vi "testpath5.vi"() -> (4 "Trajectory":T1[](array[typedef])=[{"t"=0.0, "velocity"=0.0, "acceleration"=1.0, "pose"={"Translation2d"={"x"=3.0, "y"=3.0}, "Rotation2d"={"Theta"=0.0}}, "curvature"=0.0}, {"t"=0.48107866498249907, "velocity"=0.48107866498249907, "acceleration"=1.0, "pose"={"Translation2d"={"x"=3.1157180698455615, "y"=3.0002504867135467}, "Rotation2d"={"Theta"=0.006427363502563971}}, "curvature"=0.1089996880264415}, {"t"=0.678323361711993, "velocity"=0.678323361711993, "acceleration"=1.0, "pose"={"Translation2d"={"x"=3.230048850761391, "y"=3.001918683513517}, "Rotation2d"={"Theta"=0.024668187651407807}}, "curvature"=0.20964722526020957}, {"t"=0.8269742084287445, "velocity"=0.8269742084287445, "acceleration"=1.0, "pose"={"Translation2d"={"x"=3.3418489753345284, "y"=3.006195017751254}, "Rotation2d"={"Theta"=0.05364254472795485}}, "curvature"=0.3088358096240247}, {"t"=0.9493182706582894, "velocity"=0.9493182706582894, "acceleration"=0.9999999999999989, "pose"={"Translation2d"={"x"=3.4502251031388798, "y"=3.0140362049070544}, "Rotation2d"={"Theta"=0.09263700599383605}}, "curvature"=0.4097816878257488}, {"t"=1.0541332693458725, "velocity"=1.0541332693458723, "acceleration"=1.0, "pose"={"Translation2d"={"x"=3.554516244600639, "y"=3.02618090481411}, "Rotation2d"={"Theta"=0.14101399179369137}}, "curvature"=0.512308874505636}, {"t"=1.1461185111358019, "velocity"=1.1461185111358017, "acceleration"=0.9999999999999989, "pose"={"Translation2d"={"x"=3.654276084863717, "y"=3.0431653778824543}, "Rotation2d"={"Theta"=0.19795363197982824}}, "curvature"=0.6126189634299863}, {"t"=1.2282728023077116, "velocity"=1.2282728023077114, "acceleration"=1.0, "pose"={"Translation2d"={"x"=3.7492553076551633, "y"=3.0653391413229074}, "Rotation2d"={"Theta"=0.2622253015840179}}, "curvature"=0.7032278829567145}, {"t"=1.3027431134377192, "velocity"=1.302743113437719, "acceleration"=1.0, "pose"={"Translation2d"={"x"=3.8393839191505923, "y"=3.092880625371018}, "Rotation2d"={"Theta"=0.33202347001519067}}, "curvature"=0.7738213581754176}, {"t"=1.3711828600338833, "velocity"=1.3711828600338831, "acceleration"=1.0, "pose"={"Translation2d"={"x"=3.9247535718396085, "y"=3.125812829511009}, "Rotation2d"={"Theta"=0.40492626492857636}}, "curvature"=0.8135150769014742}, {"t"=1.4349150919425286, "velocity"=1.4349150919425284, "acceleration"=1.0, "pose"={"Translation2d"={"x"=4.00559988839123, "y"=3.1640189786997217}, "Rotation2d"={"Theta"=0.4780242378088871}}, "curvature"=0.814144470711001}, {"t"=1.4950089576936443, "velocity"=1.495008957693644, "acceleration"=1.0000000000000024, "pose"={"Translation2d"={"x"=4.082284785519317, "y"=3.2072581795905597}, "Rotation2d"={"Theta"=0.5482106201854816}}, "curvature"=0.7731590788080065}, {"t"=1.5523180030026276, "velocity"=1.5523180030026276, "acceleration"=1.0, "pose"={"Translation2d"={"x"=4.1552787978479895, "y"=3.2551810767574345}, "Rotation2d"={"Theta"=0.6125488582787016}}, "curvature"=0.6945009614427361}, {"t"=1.6075049826736048, "velocity"=1.6075049826736048, "acceleration"=1.0, "pose"={"Translation2d"={"x"=4.225143401777062, "y"=3.307345508918708}, "Rotation2d"={"Theta"=0.6685937757440954}}, "curvature"=0.5870109054408447}, {"t"=1.661065404441924, "velocity"=1.661065404441924, "acceleration"=1.0, "pose"={"Translation2d"={"x"=4.29251333934746, "y"=3.363232165161137}, "Rotation2d"={"Theta"=0.714573100801571}}, "curvature"=0.46146389986649705}, {"t"=1.7133542364605543, "velocity"=1.7133542364605543, "acceleration"=1.0, "pose"={"Translation2d"={"x"=4.358078942106649, "y"=3.42226024116382}, "Rotation2d"={"Theta"=0.749411478919885}}, "curvature"=0.327879436774629}, {"t"=1.7646155759291982, "velocity"=1.7646155759291982, "acceleration"=-0.14069618652681756, "pose"={"Translation2d"={"x"=4.4225684549740585, "y"=3.4838030954221377}, "Rotation2d"={"Theta"=0.7726438166367136}}, "curvature"=0.19408566308886896}, {"t"=1.8158372909656526, "velocity"=1.7574088759562057, "acceleration"=-0.9999999999999976, "pose"={"Translation2d"={"x"=4.486730360106509, "y"=3.5472039054716995}, "Rotation2d"={"Theta"=0.7842865152488298}}, "curvature"=0.06554757707262261}, {"t"=1.8686030696202458, "velocity"=1.7046430973016127, "acceleration"=-0.9999999999999976, "pose"={"Translation2d"={"x"=4.551315700763633, "y"=3.611791324112289}, "Rotation2d"={"Theta"=0.7847207021181927}}, "curvature"=-0.05405445397664435}, {"t"=1.923774092685811, "velocity"=1.6494720742360478, "acceleration"=-1.0000000000000024, "pose"={"Translation2d"={"x"=4.617060405173301, "y"=3.6768951356318045}, "Rotation2d"={"Theta"=0.7746140906850375}}, "curvature"=-0.1620376344972609}, {"t"=1.9816328285536053, "velocity"=1.5916133383682531, "acceleration"=-0.9999999999999977, "pose"={"Translation2d"={"x"=4.684667610397049, "y"=3.741861912030208}, "Rotation2d"={"Theta"=0.7548841593229793}}, "curvature"=-0.2560779973743184}, {"t"=2.042535183657832, "velocity"=1.5307109832640264, "acceleration"=-1.0, "pose"={"Translation2d"={"x"=4.754789986195503, "y"=3.8060706692434647}, "Rotation2d"={"Theta"=0.7266900570486102}}, "curvature"=-0.3338915791528804}, {"t"=2.10694244004743, "velocity"=1.4663037268744283, "acceleration"=-1.0, "pose"={"Translation2d"={"x"=4.828012058893801, "y"=3.8689485233674916}, "Rotation2d"={"Theta"=0.6914332386010009}}, "curvature"=-0.39327428373518936}, {"t"=2.175457895843941, "velocity"=1.3977882710779173, "acceleration"=-1.000000000000001, "pose"={"Translation2d"={"x"=4.904832535247019, "y"=3.9299863468820986}, "Rotation2d"={"Theta"=0.6507460397676211}}, "curvature"=-0.4324325103085314}, {"t"=2.2488723273208384, "velocity"=1.3243738396010196, "acceleration"=-1.0, "pose"={"Translation2d"={"x"=4.9856466263055985, "y"=3.9887544248749345}, "Rotation2d"={"Theta"=0.606453056453139}}, "curvature"=-0.450438283054238}, {"t"=2.328227549017911, "velocity"=1.245018617903947, "acceleration"=-1.0, "pose"={"Translation2d"={"x"=5.070728371280769, "y"=4.044918111265431}, "Rotation2d"={"Theta"=0.5605017213985956}}, "curvature"=-0.447580511370689}, {"t"=2.414918055086827, "velocity"=1.158328111835031, "acceleration"=-1.0, "pose"={"Translation2d"={"x"=5.160212961409972, "y"=4.098253485028746}, "Rotation2d"={"Theta"=0.514872814070948}}, "curvature"=-0.4254088459788693}, {"t"=2.5108748508259513, "velocity"=1.062371316095907, "acceleration"=-0.9999999999999984, "pose"={"Translation2d"={"x"=5.254079063822289, "y"=4.148663006419709}, "Rotation2d"={"Theta"=0.4714931999649217}}, "curvature"=-0.38639049588199975}, {"t"=2.61893753775615, "velocity"=0.9543086291657085, "acceleration"=-1.0, "pose"={"Translation2d"={"x"=5.352131145403863, "y"=4.196191173196768}, "Rotation2d"={"Theta"=0.4321767854993178}}, "curvature"=-0.33325947480572066}, {"t"=2.743710613045412, "velocity"=0.8295355538764468, "acceleration"=-1.0000000000000004, "pose"={"Translation2d"={"x"=5.453981796663327, "y"=4.241040176845926}, "Rotation2d"={"Theta"=0.3986147043565599}}, "curvature"=-0.2682313688562159}, {"t"=2.893946469408784, "velocity"=0.6792996975130746, "acceleration"=-1.0000000000000002, "pose"={"Translation2d"={"x"=5.5590340555972295, "y"=4.283585558804693}, "Rotation2d"={"Theta"=0.3724265151781381}}, "curvature"=-0.1922294145483505}, {"t"=3.09198653643674, "velocity"=0.4812596304851187, "acceleration"=-0.9999999999999999, "pose"={"Translation2d"={"x"=5.666463731555449, "y"=4.324391866686028}, "Rotation2d"={"Theta"=0.35527729936540964}}, "curvature"=-0.10414472092652606}, {"t"=3.5732461669218587, "velocity"=0.0, "acceleration"=-0.9999999999999999, "pose"={"Translation2d"={"x"=5.775201729106637, "y"=4.364228310502283}, "Rotation2d"={"Theta"=0.3490658503988617}}, "curvature"=-4.0144373191817764e-15}], 6 "Reverse Path?":bool)   [LabVIEW 2019]
uses:
  AutonBuilder/Typedef/Data Point.ctl
  <vilib>/Rock Robotics/WPI/ThirdParty/WPILib Extensions/Trajectory/Typedef/Trajectory State.ctl
  <vilib>/Rock Robotics/WPI/ThirdParty/WPILib Extensions/Geometry/Typedef/Pose2d.ctl
  <vilib>/Rock Robotics/WPI/ThirdParty/WPILib Extensions/Geometry/Typedef/Translation2d.ctl
  <vilib>/Rock Robotics/WPI/ThirdParty/WPILib Extensions/Geometry/Typedef/Rotation2d.ctl
panel:
  out "Total Time (s)":dbl=3.5732461669218587
  out "Graph":cluster{dbl[], dbl[]}[](graph)=[{[2.8, 3.5, 3.5, 2.8, 2.8], [3.3, 3.3, 2.7, 2.7, 3.3]}, {[3.0, 5.775201729106628], [3.0, 4.364228310502283]}, {[3.0, 3.1157180698455615, 3.230048850761391, 3.3418489753345284, 3.4502251031388798, 3.554516244600639, 3.654276084863717, 3.7492553076551633, 3.8393839191505923, 3.9247535718396085, 4.00559988839123, 4.082284785519317, 4.1552787978479895, 4.225143401777062, 4.29251333934746, 4.358078942106649, 4.4225684549740585, 4.486730360106509, 4.551315700763633, 4.617060405173301, 4.684667610397049, 4.754789986195503, 4.828012058893801, 4.904832535247019, 4.9856466263055985, 5.070728371280769, 5.160212961409972, 5.254079063822289, 5.352131145403863, 5.453981796663327, 5.5590340555972295, 5.666463731555449, 5.775201729106637], [3.0, 3.0002504867135467, 3.001918683513517, 3.006195017751254, 3.0140362049070544, 3.02618090481411, 3.0431653778824543, 3.0653391413229074, 3.092880625371018, 3.125812829511009, 3.1640189786997217, 3.2072581795905597, 3.2551810767574345, 3.307345508918708, 3.363232165161137, 3.42226024116382, 3.4838030954221377, 3.5472039054716995, 3.611791324112289, 3.6768951356318045, 3.741861912030208, 3.8060706692434647, 3.8689485233674916, 3.9299863468820986, 3.9887544248749345, 4.044918111265431, 4.098253485028746, 4.148663006419709, 4.196191173196768, 4.241040176845926, 4.283585558804693, 4.324391866686028, 4.364228310502283]}, {[3.210100833045593, 3.1163674570857056, 3.2344256753709537, 3.35331553525211, 3.4718739962834073, 3.589216747032843, 3.7046276288946096, 3.8174590354897315, 3.9270558444895305, 4.032726350135738, 4.133780565975029, 4.229632160917573, 4.319925140468959, 4.404627655819516, 4.484052485239973, 4.558804117879396, 4.629684205195804, 4.697592968594799, 4.763451147629453, 4.828150889883975, 4.8925334632275135, 4.957387175141679, 5.023457384520475, 5.0914596639663925, 5.162086733508193, 5.236000987473815, 5.3138085081716895, 5.3960169412912, 5.482985919587022, 5.574881783592683, 5.671646985644121, 5.772990350008362, 5.878400124838382], [2.7858560298454615, 2.700251189554016, 2.7019506128687616, 2.7064142345051354, 2.7148183487794215, 2.7281945374565533, 2.7474210254195457, 2.7731949106602634, 2.805977098889792, 2.8459166359909562, 2.8927816031517377, 2.9459370151908018, 3.004399135897375, 3.066959563924363, 3.13233661390307, 3.1993041831366846, 3.266770687680612, 3.3338099966047543, 3.3996627023210784, 3.4637266406223106, 3.5255478181133677, 3.584814304292968, 3.641349919042501, 3.695102727134015, 3.7461253075572944, 3.7945484598763177, 3.8405551962975846, 3.8843646164518164, 3.926233717153275, 3.966480177646331, 4.005523824676723, 4.043942085867808, 4.082536828347791]}, {[2.789899166954407, 3.1150686826054175, 3.2256720261518286, 3.330382415416947, 3.428576209994352, 3.5198157421684346, 3.603924540832824, 3.681051579820595, 3.751711993811654, 3.8167807935434785, 3.877419210807431, 3.934937410121061, 3.9906324552270203, 4.045659147734609, 4.100974193454947, 4.157353766333901, 4.215452704752313, 4.275867751618218, 4.339180253897812, 4.405969920462626, 4.476801757566584, 4.552192797249327, 4.632566733267128, 4.7182054065276455, 4.809206519103004, 4.905455755087722, 5.006617414648254, 5.112141186353377, 5.221276371220704, 5.333081809733971, 5.446421125550338, 5.559937113102537, 5.672003333374892], [3.2141439701545385, 3.300249783873077, 3.301886754158273, 3.305975800997373, 3.3132540610346872, 3.3241672721716666, 3.338909730345363, 3.3574833719855515, 3.3797841518522445, 3.405709023031062, 3.4352563542477057, 3.4685793439903176, 3.505963017617494, 3.5477314539130527, 3.5941277164192043, 3.6452162991909556, 3.7008355031636633, 3.7605978143386447, 3.8239199459035, 3.8900636306412983, 3.958176005947048, 4.027327034193961, 4.0965471276924825, 4.1648699666301825, 4.2313835421925745, 4.295287762654543, 4.355951773759907, 4.412961396387602, 4.46614862924026, 4.515600176045521, 4.561647292932663, 4.604841647504248, 4.645919792656775]}]
  in  "Data Points":T5[](array[typedef])=[{"X"=3.0, "Y"=3.0, "Theta"=0.0, "Speed %"=0.0, "Disabled?"=FALSE}, {"X"=5.775201729106628, "Y"=4.364228310502283, "Theta"=20.0, "Speed %"=0.0, "Disabled?"=FALSE}]
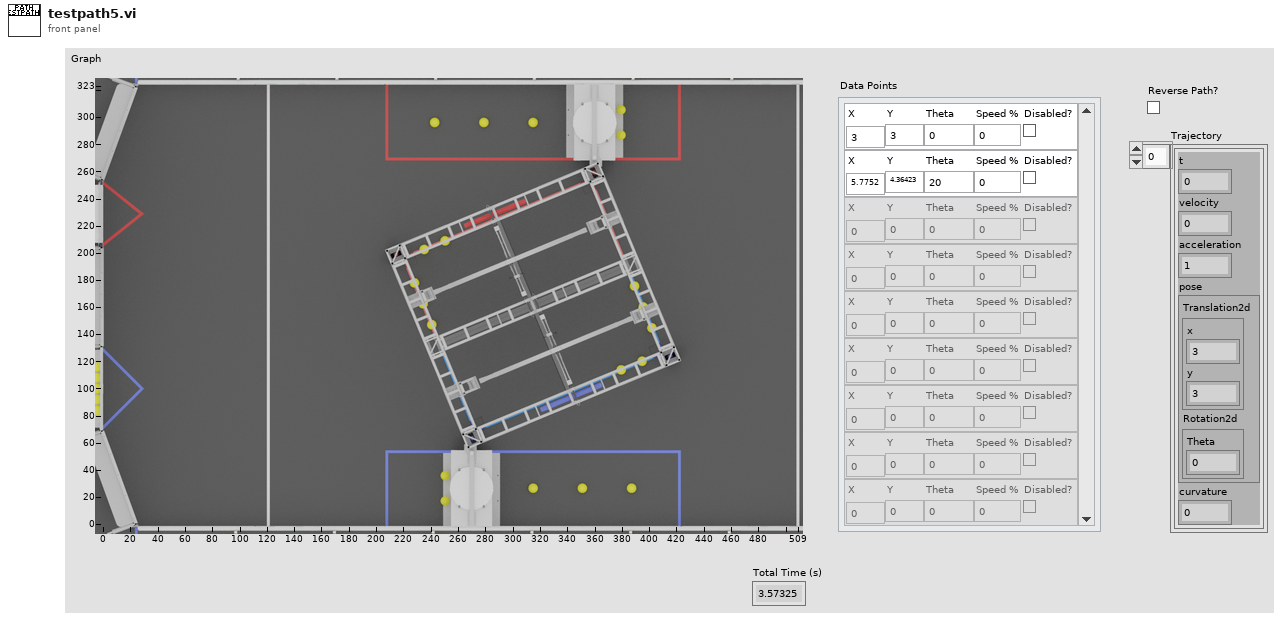
[diagram p1: front panel]
types:
  T1 = typedef "Trajectory State.ctl" = cluster{"t":dbl, "velocity":dbl, "acceleration":dbl, "pose":T2, "curvature":dbl}
  T2 = typedef "Pose2d.ctl" = cluster{"Translation2d":T3, "Rotation2d":T4}
  T3 = typedef "Translation2d.ctl" = cluster{"x":dbl, "y":dbl}
  T4 = typedef "Rotation2d.ctl" = cluster{"Theta":dbl}
  T5 = typedef "Data Point.ctl" = cluster{"X":dbl, "Y":dbl, "Theta":dbl, "Speed %":dbl, "Disabled?":bool}
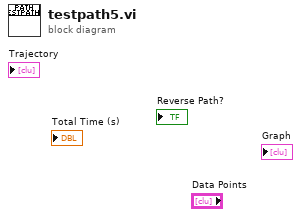
[diagram p0: block diagram]
diagram:
